vi "Server.vi"() -> ()   [LabVIEW 2023]
panel:
  in  "Tab Control":enum32{"Page 1", "Page 2", "Page 3"}(tab)
  in  "Oil tank":enum32{"Page 1"}(tab)
  out "WIndow Child Lock":bool
  out "Lock All Door":bool
  in  "Right front door":enum32{"Page 1"}(tab)
  in  "Bonnet1":enum32{"Page 1"}(tab)
  in  "Trunk1":enum32{"Page 1"}(tab)
  in  "Bonnet2":enum32{"Page 1"}(tab)
  in  "Trunk2":enum32{"Page 1"}(tab)
  in  "Right Back Door":enum32{"Page 1"}(tab)
  in  "Left Back Door":enum32{"Page 1"}(tab)
  in  "Left Front Door":enum32{"Page 1"}(tab)
  out "RFW":u8(slide) scale=0.0..100.0
  out "RBW":u8(slide) scale=0.0..100.0
  out "LBW":u8(slide) scale=0.0..100.0
  out "LFW":u8(slide) scale=0.0..100.0
  out "current time":timestamp format="%<%x>T"
  out "current time 2":timestamp format="%<%I:%M %p>T"
  in  "moonroof":enum32{"Page 1"}(tab)
  out "Low light Beam 2":bool
  out "High light Beam 2":bool
  out "Low light Beam":bool
  out "High light Beam":bool
  out "current time 4":timestamp format="%<%x>T"
  out "current time 3":timestamp format="%<%I:%M %p>T"
  out "current time 6":timestamp format="%<%x>T"
  out "current time 5":timestamp format="%<%I:%M %p>T"
  # "Left Display"
  # "Right Display"
  # "Lock All Door"
  # "Window Child Lock"
  # "Front Display"
  # "Moonroof"
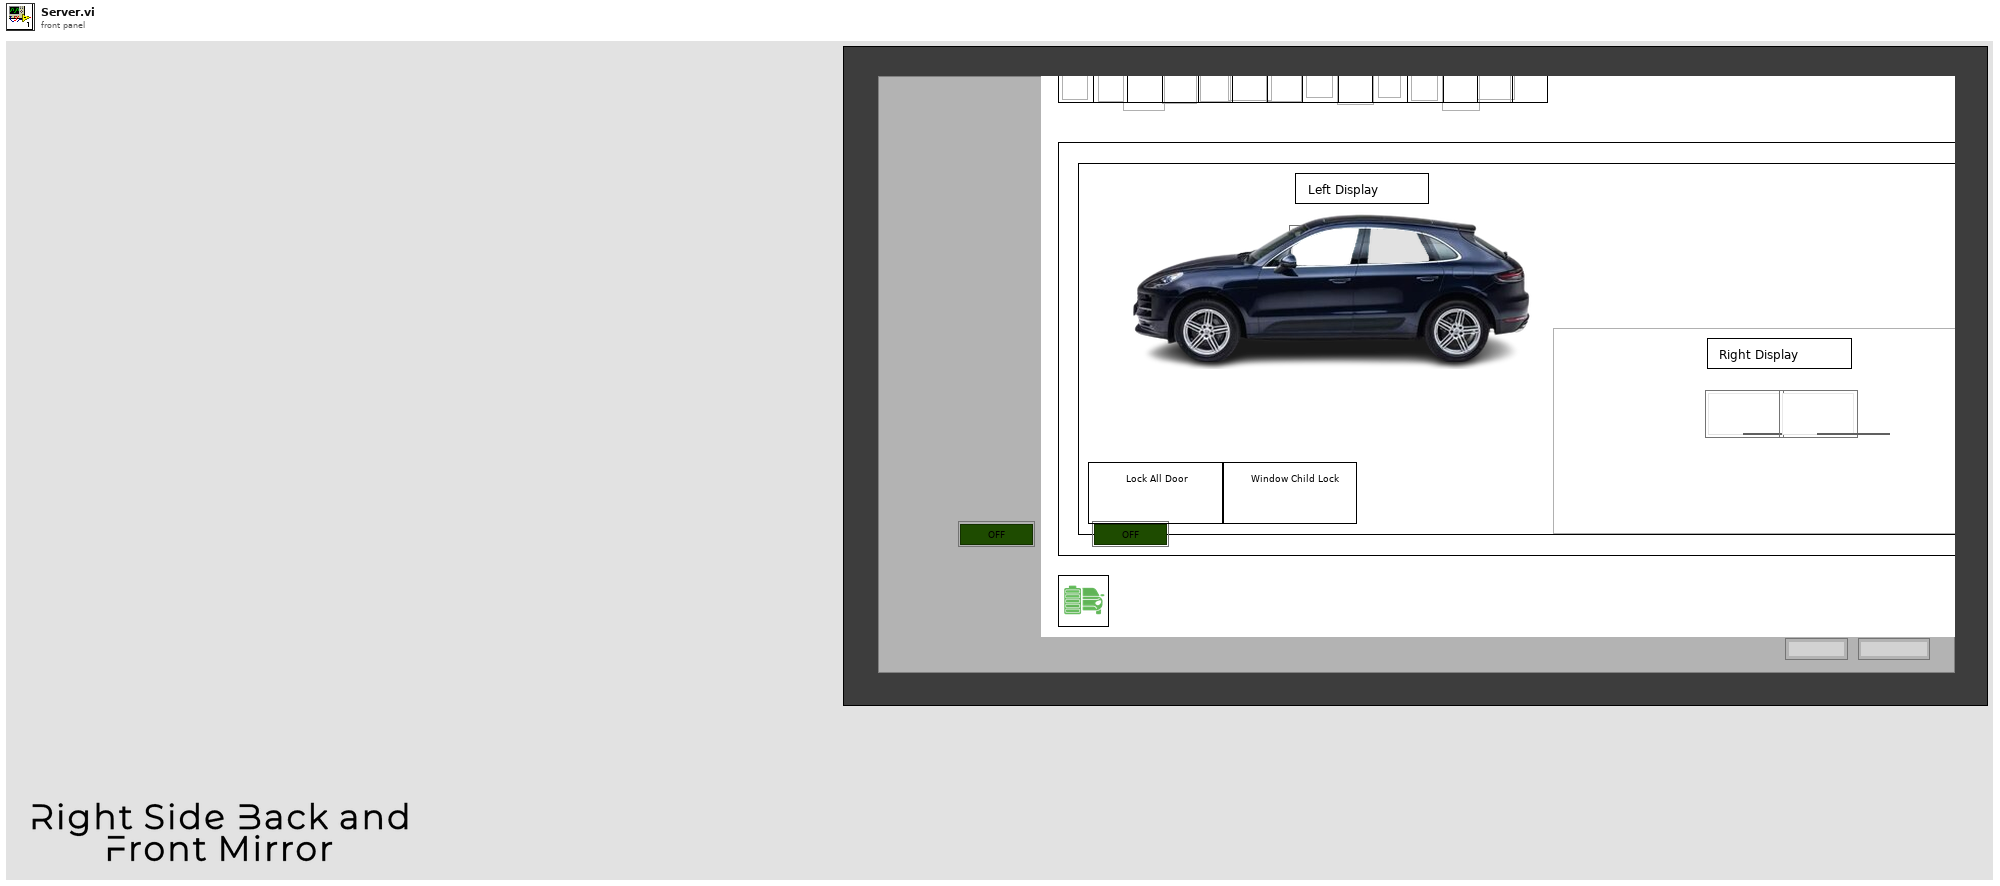
[diagram p1: front panel]
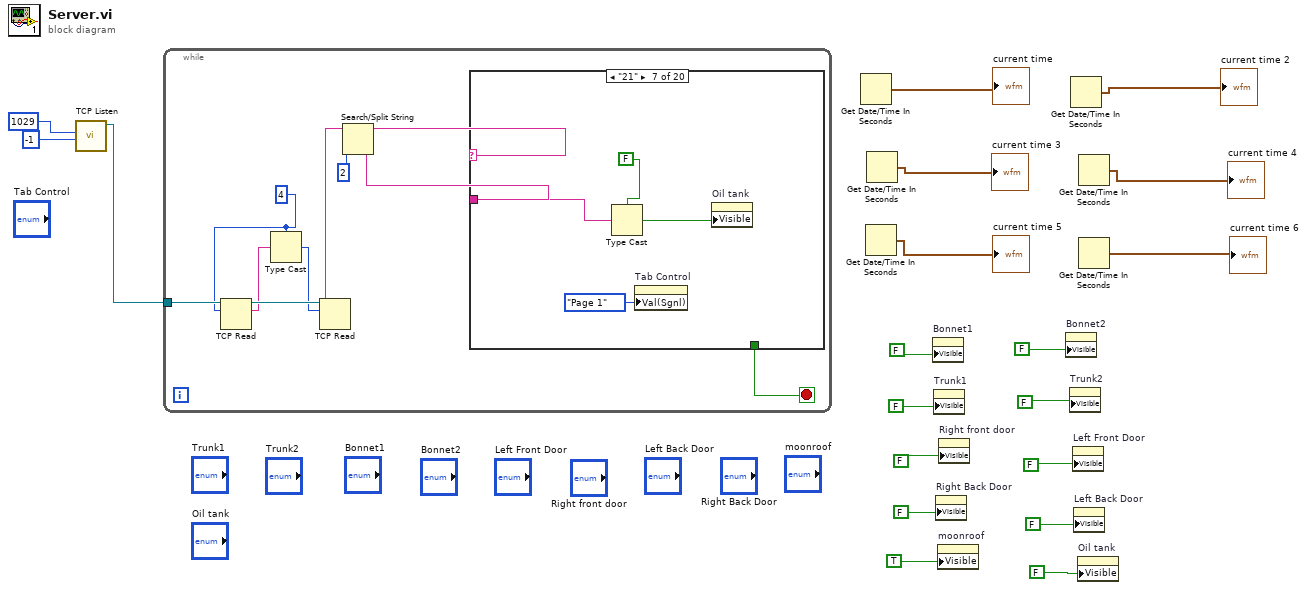
[diagram p0: block diagram]
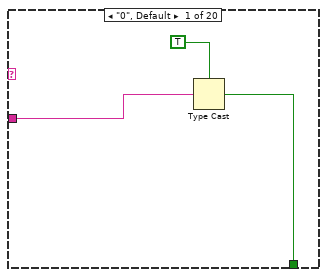
[diagram p2: hidden frame]
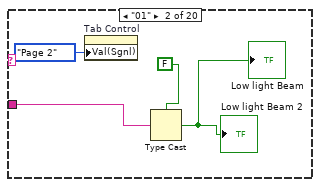
[diagram p3: hidden frame]
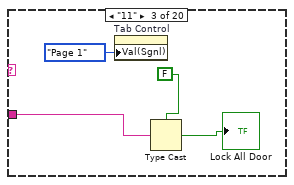
[diagram p4: hidden frame]
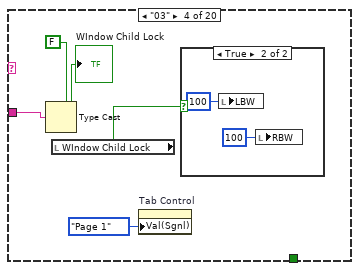
[diagram p5: hidden frame]
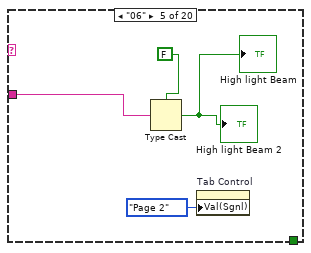
[diagram p7: hidden frame]
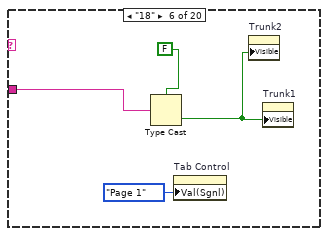
[diagram p8: hidden frame]
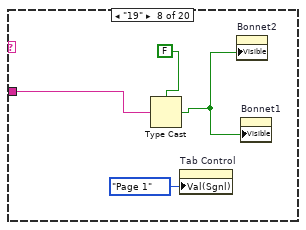
[diagram p9: hidden frame]
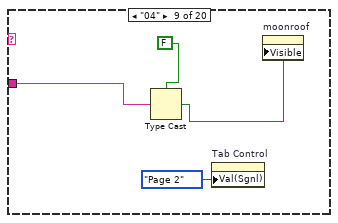
[diagram p10: hidden frame]
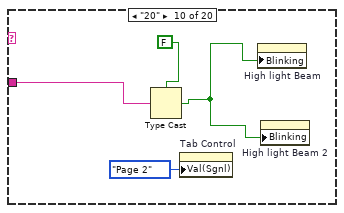
[diagram p11: hidden frame]
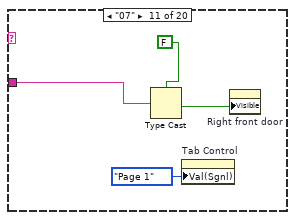
[diagram p12: hidden frame]
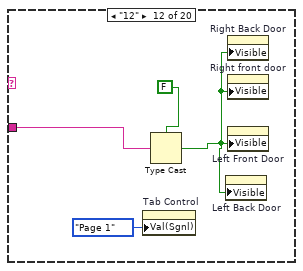
[diagram p13: hidden frame]
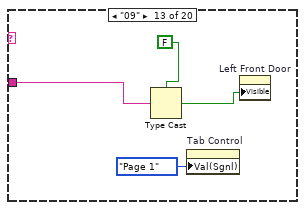
[diagram p14: hidden frame]
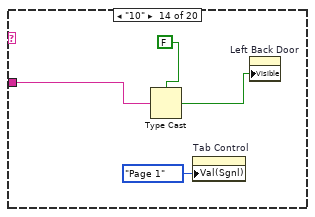
[diagram p15: hidden frame]
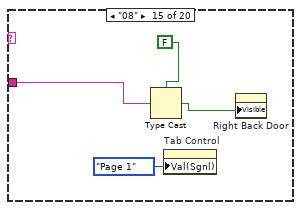
[diagram p16: hidden frame]
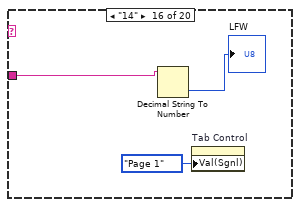
[diagram p17: hidden frame]
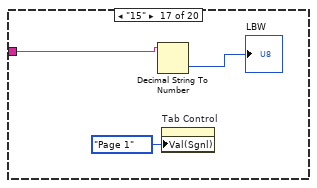
[diagram p18: hidden frame]
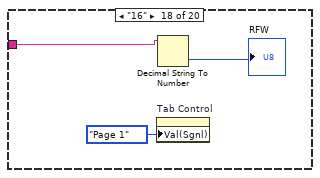
[diagram p19: hidden frame]
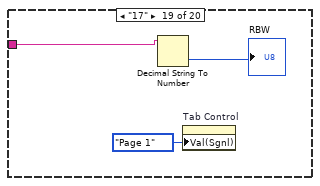
[diagram p20: hidden frame]
diagram:
  n1 = call <vilib>:"TCP Listen.vi"("timeout ms (wait forever: -1)"=-1, "port"=u16 1029) -> ("connection ID"=w17:refnum<k5>)  [unwired: 5 in, 4 out]
  n2 = while {
    tunnel: w17 -> [w29]
    stop <- w21 stop-if-true
    w26 = 4
    n3 = TCP Read(connection ID=w29, bytes to read=w26) -> (connection ID out=w28:refnum<k5>, data out=w27:string)  [unwired: 3 in, 1 out]
    n4 = Type Cast(type=w26, x=w27) -> (*(type *) &x=w23:i32)
    n5 = TCP Read(connection ID=w28, bytes to read=w23) -> (data out=w25:string)  [unwired: 3 in, 2 out]
    n6 = Search/Split String(string=w25, offset (0)=2) -> (substring before match=w20:string, match + rest of string=w22:string)  [unwired: 1 in, 1 out]
    n7 = case shown="\"21\"" w20 {
      tunnel: w22 -> [w32 w35 w39 w44 w50 w54 w58 w62 w66 w70 w74 w78 w82 w86 w90 w94 w97 w100 w103 w106]
      tunnel: [w31 _ _ _ _ _ _ _ _ _ _ _ _ _ _ _ _ _ _ _] -> w21
      frame "0", Default {
        n8 = Type Cast(type=TRUE, x=w32) -> (*(type *) &x=w31:bool)
      }
      frame "01" {
        n9 = property on="Tab Control" class="TabCtl (strict)"("Val(Sgnl)"=enum32{"Page 1", "Page 2", "Page 3"}."Page 2" ("Value (Signaling)")) -> ()  [unwired: 2 in, 2 out]
        n10 = Type Cast(type=FALSE, x=w35) -> (*(type *) &x=→"Low light Beam 2" →"Low light Beam":bool)
      }
      frame "11" {
        n11 = property on="Tab Control" class="TabCtl (strict)"("Val(Sgnl)"=enum32{"Page 1", "Page 2", "Page 3"}."Page 1" ("Value (Signaling)")) -> ()  [unwired: 2 in, 2 out]
        n12 = Type Cast(type=FALSE, x=w39) -> (*(type *) &x=→"Lock All Door":bool)
      }
      frame "03" {
        n13 = Type Cast(type=FALSE, x=w44) -> (*(type *) &x=→"WIndow Child Lock":bool)
        n14 = local read "WIndow Child Lock"() -> (w42:bool)
        n15 = property on="Tab Control" class="TabCtl (strict)"("Val(Sgnl)"=enum32{"Page 1", "Page 2", "Page 3"}."Page 1" ("Value (Signaling)")) -> ()  [unwired: 2 in, 2 out]
        n16 = case shown="True" w42 {
          frame False {
          }
          frame True {
            n17 = local write "LBW"(u8 100 ("LBW")) -> ()
            n18 = local write "RBW"(u8 100 ("RBW")) -> ()
          }
        }
      }
      frame "06" {
        n19 = Type Cast(type=FALSE, x=w50) -> (*(type *) &x=→"High light Beam 2" →"High light Beam":bool)
        n20 = property on="Tab Control" class="TabCtl (strict)"("Val(Sgnl)"=enum32{"Page 1", "Page 2", "Page 3"}."Page 2" ("Value (Signaling)")) -> ()  [unwired: 2 in, 2 out]
      }
      frame "18" {
        n21 = Type Cast(type=FALSE, x=w54) -> (*(type *) &x=w53:bool)
        n22 = property on="Tab Control" class="TabCtl (strict)"("Val(Sgnl)"=enum32{"Page 1", "Page 2", "Page 3"}."Page 1" ("Value (Signaling)")) -> ()  [unwired: 2 in, 2 out]
        n23 = property on="Trunk2" class="TabCtl (strict)"("Visible"=w53) -> ()  [unwired: 2 in, 2 out]
        n24 = property on="Trunk1" class="TabCtl (strict)"("Visible"=w53) -> ()  [unwired: 2 in, 2 out]
      }
      frame "21" {
        n25 = Type Cast(type=FALSE, x=w58) -> (*(type *) &x=w56:bool)
        n26 = property on="Tab Control" class="TabCtl (strict)"("Val(Sgnl)"=enum32{"Page 1", "Page 2", "Page 3"}."Page 1" ("Value (Signaling)")) -> ()  [unwired: 2 in, 2 out]
        n27 = property on="Oil tank" class="TabCtl (strict)"("Visible"=w56) -> ()  [unwired: 2 in, 2 out]
      }
      frame "19" {
        n28 = Type Cast(type=FALSE, x=w62) -> (*(type *) &x=w61:bool)
        n29 = property on="Tab Control" class="TabCtl (strict)"("Val(Sgnl)"=enum32{"Page 1", "Page 2", "Page 3"}."Page 1" ("Value (Signaling)")) -> ()  [unwired: 2 in, 2 out]
        n30 = property on="Bonnet2" class="TabCtl (strict)"("Visible"=w61) -> ()  [unwired: 2 in, 2 out]
        n31 = property on="Bonnet1" class="TabCtl (strict)"("Visible"=w61) -> ()  [unwired: 2 in, 2 out]
      }
      frame "04" {
        n32 = Type Cast(type=FALSE, x=w66) -> (*(type *) &x=w65:bool)
        n33 = property on="Tab Control" class="TabCtl (strict)"("Val(Sgnl)"=enum32{"Page 1", "Page 2", "Page 3"}."Page 2" ("Value (Signaling)")) -> ()  [unwired: 2 in, 2 out]
        n34 = property on="moonroof" class="TabCtl (strict)"("Visible"=w65) -> ()  [unwired: 2 in, 2 out]
      }
      frame "20" {
        n35 = Type Cast(type=FALSE, x=w70) -> (*(type *) &x=w69:bool)
        n36 = property on="Tab Control" class="TabCtl (strict)"("Val(Sgnl)"=enum32{"Page 1", "Page 2", "Page 3"}."Page 2" ("Value (Signaling)")) -> ()  [unwired: 2 in, 2 out]
        n37 = property on="High light Beam" class="Bool (strict)"("Blinking"=w69) -> ()  [unwired: 2 in, 2 out]
        n38 = property on="High light Beam 2" class="Bool (strict)"("Blinking"=w69) -> ()  [unwired: 2 in, 2 out]
      }
      frame "07" {
        n39 = Type Cast(type=FALSE, x=w74) -> (*(type *) &x=w73:bool)
        n40 = property on="Tab Control" class="TabCtl (strict)"("Val(Sgnl)"=enum32{"Page 1", "Page 2", "Page 3"}."Page 1" ("Value (Signaling)")) -> ()  [unwired: 2 in, 2 out]
        n41 = property on="Right front door" class="TabCtl (strict)"("Visible"=w73) -> ()  [unwired: 2 in, 2 out]
      }
      frame "12" {
        n42 = property on="Tab Control" class="TabCtl (strict)"("Val(Sgnl)"=enum32{"Page 1", "Page 2", "Page 3"}."Page 1" ("Value (Signaling)")) -> ()  [unwired: 2 in, 2 out]
        n43 = Type Cast(type=FALSE, x=w78) -> (*(type *) &x=w77:bool)
        n44 = property on="Left Back Door" class="TabCtl (strict)"("Visible"=w77) -> ()  [unwired: 2 in, 2 out]
        n45 = property on="Right Back Door" class="TabCtl (strict)"("Visible"=w77) -> ()  [unwired: 2 in, 2 out]
        n46 = property on="Right front door" class="TabCtl (strict)"("Visible"=w77) -> ()  [unwired: 2 in, 2 out]
        n47 = property on="Left Front Door" class="TabCtl (strict)"("Visible"=w77) -> ()  [unwired: 2 in, 2 out]
      }
      frame "09" {
        n48 = Type Cast(type=FALSE, x=w82) -> (*(type *) &x=w81:bool)
        n49 = property on="Tab Control" class="TabCtl (strict)"("Val(Sgnl)"=enum32{"Page 1", "Page 2", "Page 3"}."Page 1" ("Value (Signaling)")) -> ()  [unwired: 2 in, 2 out]
        n50 = property on="Left Front Door" class="TabCtl (strict)"("Visible"=w81) -> ()  [unwired: 2 in, 2 out]
      }
      frame "10" {
        n51 = Type Cast(type=FALSE, x=w86) -> (*(type *) &x=w85:bool)
        n52 = property on="Tab Control" class="TabCtl (strict)"("Val(Sgnl)"=enum32{"Page 1", "Page 2", "Page 3"}."Page 1" ("Value (Signaling)")) -> ()  [unwired: 2 in, 2 out]
        n53 = property on="Left Back Door" class="TabCtl (strict)"("Visible"=w85) -> ()  [unwired: 2 in, 2 out]
      }
      frame "08" {
        n54 = Type Cast(type=FALSE, x=w90) -> (*(type *) &x=w89:bool)
        n55 = property on="Tab Control" class="TabCtl (strict)"("Val(Sgnl)"=enum32{"Page 1", "Page 2", "Page 3"}."Page 1" ("Value (Signaling)")) -> ()  [unwired: 2 in, 2 out]
        n56 = property on="Right Back Door" class="TabCtl (strict)"("Visible"=w89) -> ()  [unwired: 2 in, 2 out]
      }
      frame "14" {
        n57 = Decimal String To Number(string=w94) -> (number=→"LFW":i32)  [unwired: 2 in, 1 out]
        n58 = property on="Tab Control" class="TabCtl (strict)"("Val(Sgnl)"=enum32{"Page 1", "Page 2", "Page 3"}."Page 1" ("Value (Signaling)")) -> ()  [unwired: 2 in, 2 out]
      }
      frame "15" {
        n59 = Decimal String To Number(string=w97) -> (number=→"LBW":i32)  [unwired: 2 in, 1 out]
        n60 = property on="Tab Control" class="TabCtl (strict)"("Val(Sgnl)"=enum32{"Page 1", "Page 2", "Page 3"}."Page 1" ("Value (Signaling)")) -> ()  [unwired: 2 in, 2 out]
      }
      frame "16" {
        n61 = property on="Tab Control" class="TabCtl (strict)"("Val(Sgnl)"=enum32{"Page 1", "Page 2", "Page 3"}."Page 1" ("Value (Signaling)")) -> ()  [unwired: 2 in, 2 out]
        n62 = Decimal String To Number(string=w100) -> (number=→"RFW":i32)  [unwired: 2 in, 1 out]
      }
      frame "17" {
        n63 = Decimal String To Number(string=w103) -> (number=→"RBW":i32)  [unwired: 2 in, 1 out]
        n64 = property on="Tab Control" class="TabCtl (strict)"("Val(Sgnl)"=enum32{"Page 1", "Page 2", "Page 3"}."Page 1" ("Value (Signaling)")) -> ()  [unwired: 2 in, 2 out]
      }
      frame "02" {
        n65 = property on="Tab Control" class="TabCtl (strict)"("Val(Sgnl)"=enum32{"Page 1", "Page 2", "Page 3"}."Page 1" ("Value (Signaling)")) -> ()  [unwired: 2 in, 2 out]
        n66 = Type Cast(type=FALSE, x=w106) -> (*(type *) &x=w105:bool)
        n67 = case shown="False" w105 {
          frame True {
            w108 = u8 0 ("RBW 2")
            n68 = local write "RBW"(w108) -> ()
            n69 = local write "RFW"(w108) -> ()
            n70 = local write "LBW"(w108) -> ()
            n71 = local write "LFW"(w108) -> ()
          }
          frame False {
            w109 = u8 100 ("RBW 2")
            n72 = local write "RBW"(w109) -> ()
            n73 = local write "RFW"(w109) -> ()
            n74 = local write "LBW"(w109) -> ()
            n75 = local write "LFW"(w109) -> ()
          }
        }
      }
    }
  }
  n76 = Get Date/Time In Seconds() -> (seconds since 1Jan1904=→"current time":timestamp)
  n77 = Get Date/Time In Seconds() -> (seconds since 1Jan1904=→"current time 5":timestamp)
  n78 = Get Date/Time In Seconds() -> (seconds since 1Jan1904=→"current time 3":timestamp)
  n79 = property on="Bonnet1" class="TabCtl (strict)"("Visible"=FALSE) -> ()  [unwired: 2 in, 2 out]
  n80 = property on="Trunk1" class="TabCtl (strict)"("Visible"=FALSE) -> ()  [unwired: 2 in, 2 out]
  n81 = property on="Right Back Door" class="TabCtl (strict)"("Visible"=FALSE) -> ()  [unwired: 2 in, 2 out]
  n82 = property on="moonroof" class="TabCtl (strict)"("Visible"=TRUE) -> ()  [unwired: 2 in, 2 out]
  n83 = property on="Right front door" class="TabCtl (strict)"("Visible"=FALSE) -> ()  [unwired: 2 in, 2 out]
  n84 = property on="Bonnet2" class="TabCtl (strict)"("Visible"=FALSE) -> ()  [unwired: 2 in, 2 out]
  n85 = property on="Trunk2" class="TabCtl (strict)"("Visible"=FALSE) -> ()  [unwired: 2 in, 2 out]
  n86 = Get Date/Time In Seconds() -> (seconds since 1Jan1904=→"current time 2":timestamp)
  n87 = property on="Left Front Door" class="TabCtl (strict)"("Visible"=FALSE) -> ()  [unwired: 2 in, 2 out]
  n88 = property on="Left Back Door" class="TabCtl (strict)"("Visible"=FALSE) -> ()  [unwired: 2 in, 2 out]
  n89 = property on="Oil tank" class="TabCtl (strict)"("Visible"=FALSE) -> ()  [unwired: 2 in, 2 out]
  n90 = Get Date/Time In Seconds() -> (seconds since 1Jan1904=→"current time 4":timestamp)
  n91 = Get Date/Time In Seconds() -> (seconds since 1Jan1904=→"current time 6":timestamp)
